vi "WriteCal.vi"(8 "Password":string, 9 "Valor de control sobrecarga:":u16, 10 "Unidades":u8(ring) items=["Kg", "N", "Lb"], 11 "Captador":u8(ring) caption="Captador utilizado:" items=["Célula 2000 Kg", "Célula Adicional"]) -> ()   [LabVIEW 2014]
uses:
  <vilib>/registry/registry.llb/Registry RtKey.ctl
  <vilib>/registry/registry.llb/Write Registry Value Simple STR.vi
  <vilib>/SEA/LTK/LTK_API.lvlib
panel:
  in  "error in (no error)":errorcluster
  out "error out":errorcluster
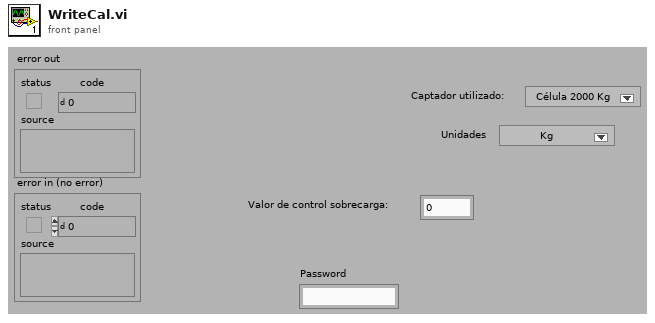
[diagram p1: front panel]
types:
  T1 = typedef "Registry RtKey.ctl" = enum32{"HKEY_CLASSES_ROOT", "HKEY_CURRENT_USER", "HKEY_LOCAL_MACHINE", "HKEY_USERS", "HKEY_PERFORMANCE_DATA", "HKEY_CURRENT_CONFIG", "HKEY_DYN_DATA"}
  T2 = typedef "Registry refnum.ctl" = refnum<k1>
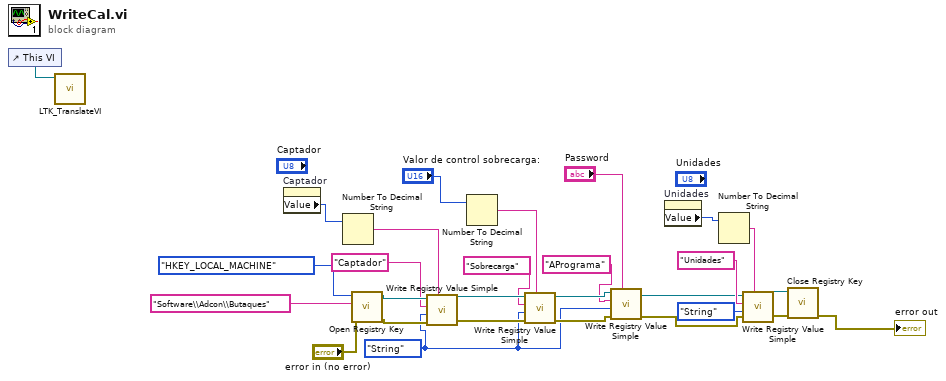
[diagram p0: block diagram]
diagram:
  w3 = enum16{"String", "Binary", "DWORD"}."String" ("simple data type")
  n1 = control-ref of="This VI"() -> (w1:refnum<vi>)
  n2 = call <vilib>:"LTK_TranslateVI.vi"("VIRef"=w1) -> ()  [unwired: 10 in, 1 out]
  n3 = property on="Captador" class="Ring (strict)"() -> ("Value"=w18:u8)  [unwired: 2 in, 2 out]
  n4 = Number To Decimal String(number=w18) -> (decimal integer string=w12:string)  [unwired: 1 in]
  n5 = call <vilib>:"Open Registry Key.vi"("error in (no error)"="error in (no error)", "subkey"="Software\\Adcon\\Butaques", "root key (HKEY_LOCAL_MACHINE)"=Registry_RtKey."HKEY_LOCAL_MACHINE") -> ("error out"=w20:errorcluster, "refnum out"=w21:T2)  [unwired: 7 in]
  n6 = call-poly <vilib>:"Write Registry Value Simple.vi"("String/Binary data"=w12, "error in (no error)"=w20, "simple data type"=w3, "value"="Captador", "refnum"=w21) -> ("error out"=w22:errorcluster, "refnum out"=w23:T2)  [unwired: 3 in]
  n7 = Number To Decimal String(number="Valor de control sobrecarga:") -> (decimal integer string=w14:string)  [unwired: 1 in]
  n8 = call-poly <vilib>:"Write Registry Value Simple.vi"("String/Binary data"=w14, "error in (no error)"=w22, "simple data type"=w3, "value"="Sobrecarga", "refnum"=w23) -> ("error out"=w8:errorcluster, "refnum out"=w5:T2)  [unwired: 3 in]
  n9 = call-poly <vilib>:"Write Registry Value Simple.vi"("String/Binary data"="Password", "error in (no error)"=w8, "simple data type"=w3, "value"="APrograma", "refnum"=w5) -> ("error out"=w7:errorcluster, "refnum out"=w6:T2)  [unwired: 3 in]
  n10 = property on="Unidades" class="Ring (strict)"() -> ("Value"=w16:u8)  [unwired: 2 in, 2 out]
  n11 = Number To Decimal String(number=w16) -> (decimal integer string=w10:string)  [unwired: 1 in]
  n12 = call-poly <vilib>:"Write Registry Value Simple.vi"("String/Binary data"=w10, "error in (no error)"=w7, "simple data type"=enum16{"String", "Binary", "DWORD"}."String", "value"="Unidades", "refnum"=w6) -> ("error out"=w24:errorcluster, "refnum out"=w19:T2)  [unwired: 3 in]
  n13 = call <vilib>:"Close Registry Key.vi"("error in (no error)"=w24, "refnum"=w19) -> ("error out"=→"error out":errorcluster)  [unwired: 5 in]
